vi "Controller - Perform DAQ Data.vi"(8 "error in (no error)":errorcluster, 10 "RT Data portion":dbl[](array[numeric]), 11 "View Model":T1) -> (0 "error out":errorcluster, 3 "View Model":T1)   [LabVIEW 2017]
doc: "This SubVI perform DAQ data from RT Data portion before saving to TDMS."
uses:
  View Model/Controls/View Model.ctl
  View Model/Controls/Shared Model.ctl
  Error Handler/Controls/Error Model.ctl
  Error Handler/Controls/Error Event.ctl
  Error Handler/Controls/Error Type.ctl
  Controls/Controller Model.ctl
  Controls/Controller Event.ctl
  Controls/Controller Command.ctl
  Controls/Controller Overhead.ctl
  Real-Time/RT Status.ctl
  Real-Time/RT Loop Status.ctl
  Controls/Controller NStream.ctl
  Controls/Controller DAQ Data.ctl
  TDMS Logger/Controls/TDMS Model.ctl
  TDMS Logger/Controls/TDMS Event.ctl
  TDMS Logger/Controls/TDMS Command.ctl
  TDMS Logger/Controls/TDMS Overhead.ctl
  TDMS Logger/Controls/TDMS ChanProperties.ctl
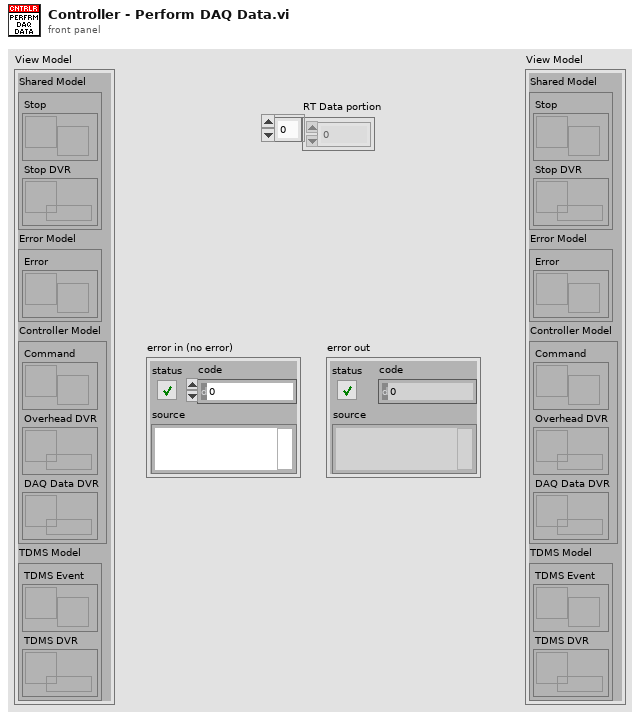
[diagram p1: front panel]
types:
  T1 = typedef "View Model.ctl" = cluster{"Shared Model":T2, "Error Model":T3, "Controller Model":T4, "TDMS Model":T5}
  T2 = typedef "Shared Model.ctl" = cluster{"Stop":refnum<user-event>, "Stop DVR":refnum<data-value>}
  T3 = typedef "Error Model.ctl" = cluster{"Error":refnum<user-event>}
  T4 = typedef "Controller Model.ctl" = cluster{"Command":refnum<user-event>, "Overhead DVR":refnum<data-value>, "DAQ Data DVR":refnum<data-value>}
  T5 = typedef "TDMS Model.ctl" = cluster{"TDMS Event":refnum<user-event>, "TDMS DVR":refnum<data-value>}
  T6 = typedef "Controller DAQ Data.ctl" = cluster{"AOM data":dbl[], "AIMV data":dbl[], "AIMC data":dbl[], "DOM data":dbl[], "DIM data":dbl[], "AOM timestamp":dbl, "AIMV timestamp":dbl, "AIMC timestamp":dbl, "DOM timestamp":dbl, "DIM timestamp":dbl}
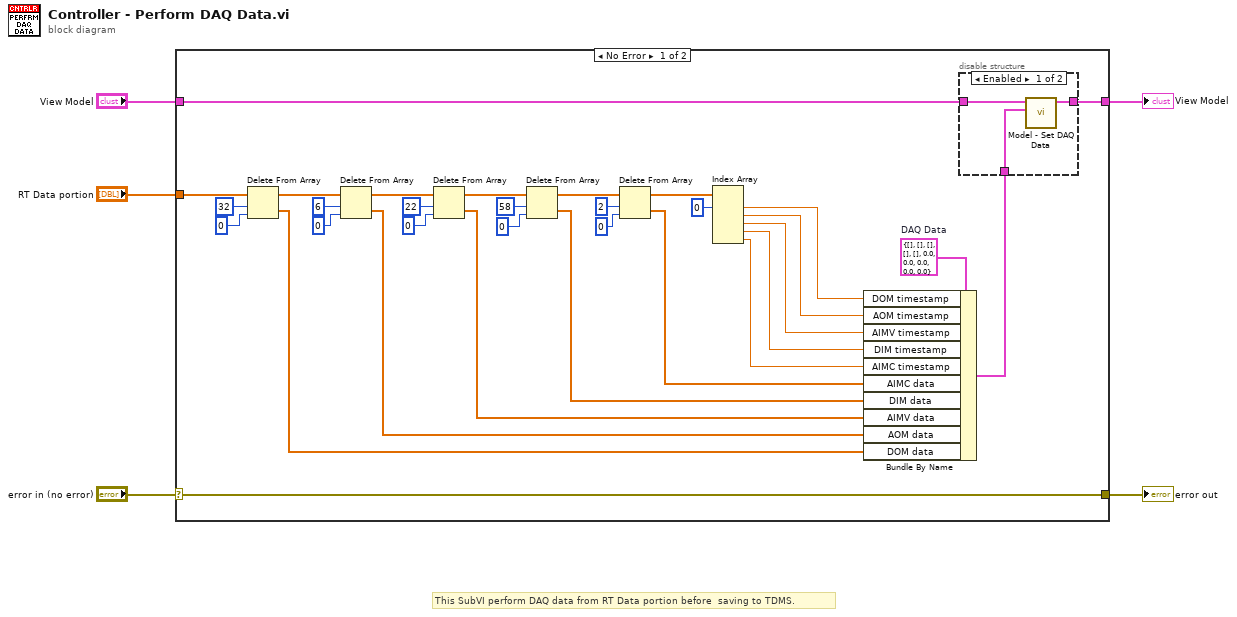
[diagram p0: block diagram]
diagram:
  # "This SubVI perform DAQ data from RT Data portion before  saving to TDMS."
  n1 = case shown="No Error" "error in (no error)" {
    selector: "error in (no error)" -> [w37 w42]
    tunnel: [w37 w42] -> w4
    tunnel: "View Model" -> [w35 w43]
    tunnel: [w34 w43] -> w2
    tunnel: "RT Data portion" -> [w6 _]
    frame No Error {
      w36 = T6 {"AOM data"=[], "AIMV data"=[], "AIMC data"=[], "DOM data"=[], "DIM data"=[], "AOM timestamp"=0.0, "AIMV timestamp"=0.0, "AIMC timestamp"=0.0, "DOM timestamp"=0.0, "DIM timestamp"=0.0}  # DAQ Data
      n2 = Delete From Array(array=w6, length=32, index=0) -> (deleted portion=w30:dbl[], array with subset deleted=w29:dbl[])
      n3 = Delete From Array(array=w29, length=6, index=0) -> (deleted portion=w26:dbl[], array with subset deleted=w25:dbl[])
      n4 = Delete From Array(array=w25, length=22, index=0) -> (deleted portion=w22:dbl[], array with subset deleted=w19:dbl[])
      n5 = Delete From Array(array=w19, length=58, index=0) -> (deleted portion=w18:dbl[], array with subset deleted=w15:dbl[])
      n6 = Delete From Array(array=w15, length=2, index=0) -> (deleted portion=w14:dbl[], array with subset deleted=w7:dbl[])
      n7 = Index Array(array=w7, index #1=0 ("index")) -> (element #1=w8:dbl, element #2=w9:dbl, element #3=w10:dbl, element #4=w11:dbl, element #5=w12:dbl)  [unwired: 4 in]
      n8 = Bundle By Name(cluster=w36, "DOM timestamp"=w8, "AOM timestamp"=w9, "AIMV timestamp"=w10, "DIM timestamp"=w11, "AIMC timestamp"=w12, "AIMC data"=w14, "DIM data"=w18, "AIMV data"=w22, "AOM data"=w26, "DOM data"=w30) -> (w33:T6)
      n9 = disable-structure shown="Enabled" {
        disable-tunnel: w35 -> [w40 w41]
        disable-tunnel: [w39 w41] -> w34
        disable-tunnel: w33 -> [w38 _]
        frame Enabled {
          n10 = call "Model - Set DAQ Data.vi"("DAQ Data"=w38, "View Model"=w40) -> ("View Model"=w39:T1)  [unwired: 8 in, 1 out]
        }
        frame Disabled {
        }
      }
    }
    frame Error {
    }
  }
  "View Model" <- w2
  "error out" <- w4
